vi "dfd_Weighted LSE Solution.vi"   [LabVIEW 2017, in "NI_DigFilter_Design.lvlib"]
uses:
  <vilib>/addons/Digital Filter Design/NI_DigFilter_Design.lvlib
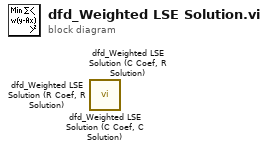
[diagram p0: block diagram]
diagram:
  n1 = call <vilib>:"dfd_Weighted LSE Solution (C Coef, C Solution).vi"() -> ()  [unwired: 9 in, 3 out]
  n2 = call <vilib>:"dfd_Weighted LSE Solution (C Coef, R Solution).vi"() -> ()  [unwired: 9 in, 3 out]
  n3 = call <vilib>:"dfd_Weighted LSE Solution (R Coef, R Solution).vi"() -> ()  [unwired: 9 in, 3 out]
